vi "Param limits calc.vi"(6 "control":T1={"GAIN"=1.0, "OFFSET"=0.0, "TIME_CONST"=100.0, "MINOFFSET"=2.0, "PVMIN"=0.0, "MINACC"=0.0, "LL"=1.0, "L"=2.0, "H"=6.0, "HH"=7.0, "MAXACC"=9.0, "PVMAX"=10.0, "MAXOFFSET"=2.0, "D"=0.5, "VMAX"=0.0, "TOUT"=1.0, "APERTURE"=0.0} {"APERTURE" min=-100000.0 max=100000.0 step=0.0010000000474974513; "TOUT" min=0.0 max=100000.0 step=1.0; "D" min=-100000.0 max=100000.0 step=0.0010000000474974513; "MAXOFFSET" min=0.0 max=50.0 step=0.0010000000474974513; "PVMAX" min=-100000.0 max=100000.0 step=0.0010000000474974513; "MAXACC" min=-100000.0 max=100000.0 step=0.0010000000474974513; "HH" min=-100000.0 max=100000.0 step=0.0010000000474974513; "H" min=-100000.0 max=100000.0 step=0.0010000000474974513; "L" min=-100000.0 max=100000.0 step=0.0010000000474974513; "LL" min=-100000.0 max=100000.0 step=0.0010000000474974513; "MINACC" min=-100000.0 max=100000.0 step=0.0010000000474974513; "PVMIN" min=-100000.0 max=100000.0 step=0.0010000000474974513; "MINOFFSET" min=0.0 max=50.0 step=0.0010000000474974513; "TIME_CONST" min=1.0 max=100000.0 step=1.0; "OFFSET" min=-100000.0 max=100000.0 step=0.0010000000474974513; "GAIN" min=0.0010000000474974513 max=1000.0 step=0.0010000000474974513}, 7 "PV":dbl step=0.009999999776482582) -> (0 "block":u32 format="%09b", 1 "Off":u32 format="%09b", 2 "On":u32 format="%09b", 3 "PVOUT":dbl format="%#_3g")   [LabVIEW 2019, in "Inputs.lvlib"]
uses:
  Inputs.lvlib
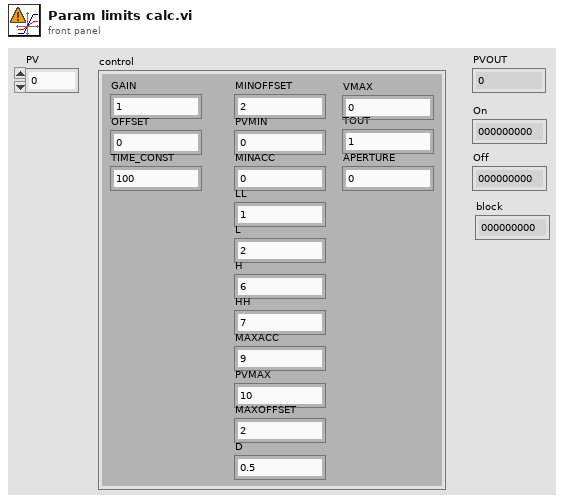
[diagram p1: front panel]
types:
  T1 = cluster{"GAIN":dbl, "OFFSET":dbl, "TIME_CONST":dbl, "MINOFFSET":dbl, "PVMIN":dbl, "MINACC":dbl, "LL":dbl, "L":dbl, "H":dbl, "HH":dbl, "MAXACC":dbl, "PVMAX":dbl, "MAXOFFSET":dbl, "D":dbl, "VMAX":dbl, "TOUT":dbl, "APERTURE":dbl}
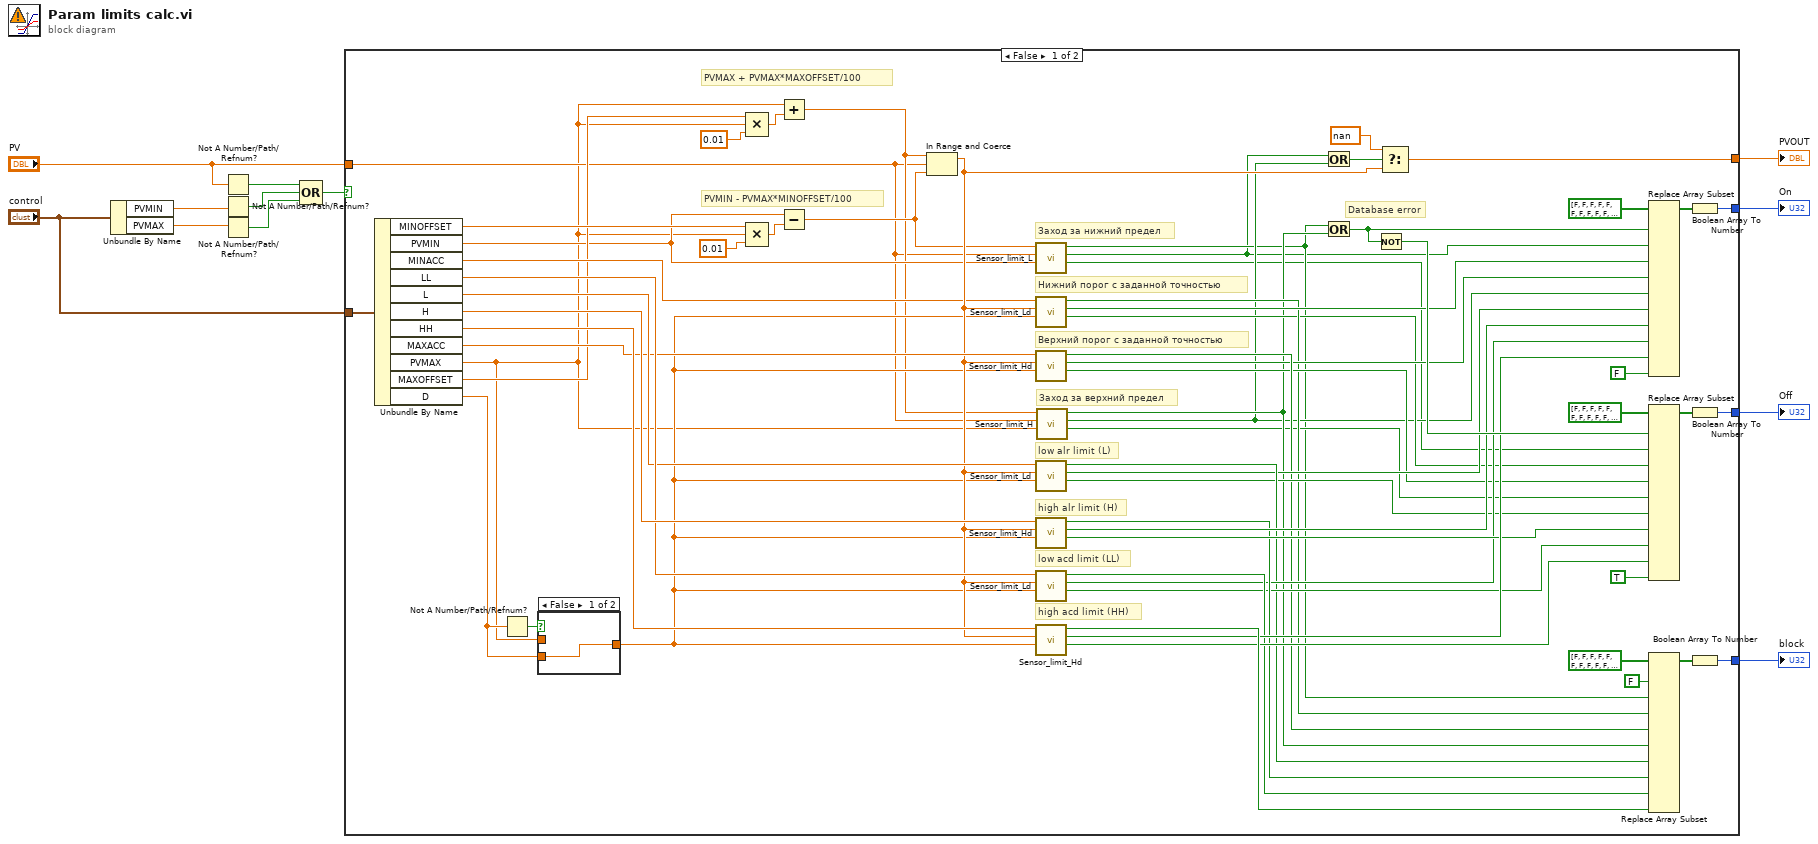
[diagram p0: block diagram]
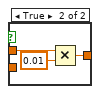
[diagram p2: hidden frame]
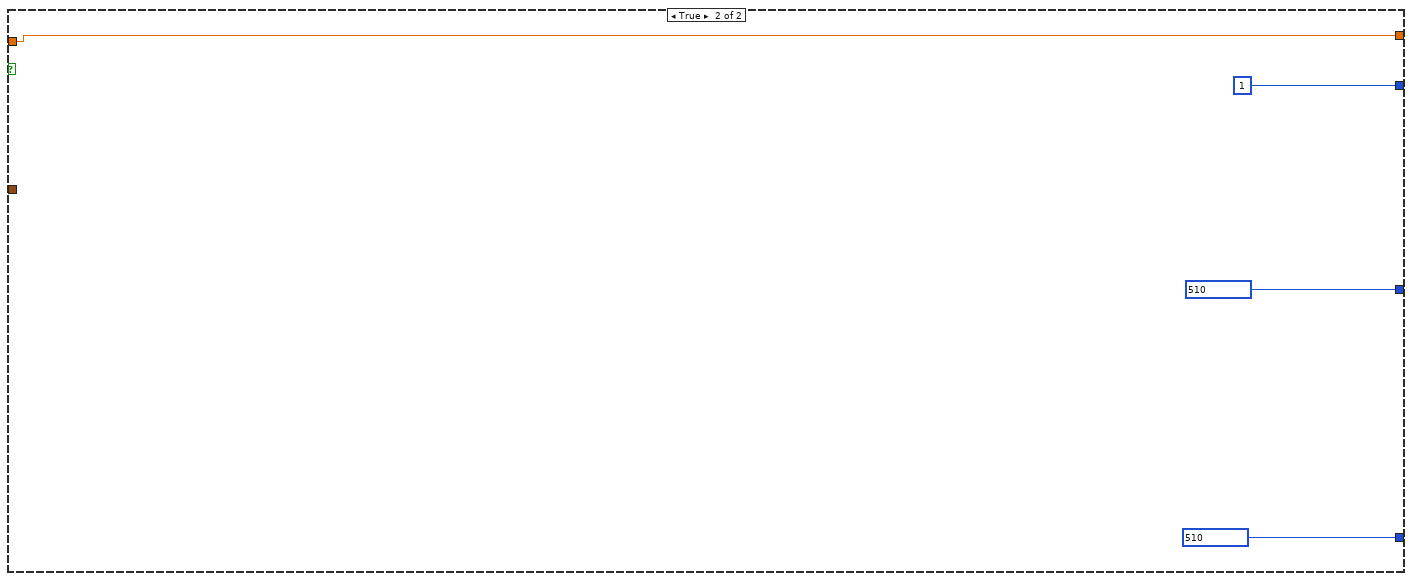
[diagram p3: hidden frame]
diagram:
  n1 = Unbundle By Name("control") -> ("PVMIN"=w10:dbl, "PVMAX"=w9:dbl)
  n2 = Not A Number/Path/Refnum?(number/path/refnum="PV") -> (NaN/Path/Refnum?=w8:bool)
  n3 = Not A Number/Path/Refnum?(number/path/refnum=w10) -> (NaN/Path/Refnum?=w12:bool)
  n4 = Not A Number/Path/Refnum?(number/path/refnum=w9) -> (NaN/Path/Refnum?=w11:bool)
  n5 = Compound Arithmetic op=OR(w8, w12, w11) -> (w6:bool)
  n6 = case shown="False" w6 {
    tunnel: [w72 w83] -> w4
    tunnel: "PV" -> [w17 w83]
    tunnel: [w62 u32 1] -> w3
    tunnel: [w65 u32 510] -> w2
    tunnel: "control" -> [w75 _]
    tunnel: [w74 u32 510] -> w1
    frame False {
      # "Database error"
      # "Верхний порог с заданной точностью"
      # "high acd limit (HH)"
      # "high alr limit (H)"
      # "low acd limit (LL)"
      # "low alr limit (L)"
      # "Заход за верхний предел"
      # "Нижний порог с заданной точностью"
      # "Заход за нижний предел"
      # "PVMIN - PVMAX*MINOFFSET/100"
      # "PVMAX + PVMAX*MAXOFFSET/100"
      n7 = Unbundle By Name(w75) -> ("MINOFFSET"=w60:dbl, "PVMIN"=w20:dbl, "MINACC"=w30:dbl, "LL"=w46:dbl, "L"=w42:dbl, "H"=w50:dbl, "HH"=w54:dbl, "MAXACC"=w36:dbl, "PVMAX"=w13:dbl, "MAXOFFSET"=w23:dbl, "D"=w38:dbl)
      n8 = Not A Number/Path/Refnum?(number/path/refnum=w38) -> (NaN/Path/Refnum?=w37:bool)
      n9 = case shown="False" w37 {
        tunnel: w13 -> [_ w78]
        tunnel: [w76 w77] -> w31
        tunnel: w38 -> [w76 _]
        frame False {
        }
        frame True {
          n10 = Multiply(x=w78, y=0.01) -> (x*y=w77:dbl)
        }
      }
      n11 = Compound Arithmetic op=MULTIPLY(w23, w13, 0.01 ("value")) -> (w21:dbl)
      n12 = Compound Arithmetic op=MULTIPLY(w60, w13, 0.01 ("value")) -> (w59:dbl)
      n13 = Add(x=w13, y=w21) -> (x+y=w18:dbl)
      n14 = Subtract(x=w20, y=w59) -> (x-y=w19:dbl)
      n15 = In Range and Coerce(upper limit=w18, x=w17, lower limit=w19) -> (coerced(x)=w32:dbl)  [unwired: 1 out]
      n16 = call "Sensor_limit_L.vi"("Off L"=w20, "PV"=w17, "Limit L"=w19) -> ("Off"=w14:bool, "On"=w15:bool, "NaN"=w16:bool)  [unwired: 6 in]
      n17 = call "Sensor_limit_Ld.vi"("d"=w31, "PV"=w32, "Limit L"=w30) -> ("Off"=w27:bool, "On"=w29:bool, "NaN"=w28:bool)  [unwired: 6 in]
      n18 = call "Sensor_limit_Hd.vi"("d"=w31, "PV"=w32, "Limit H"=w36) -> ("Off"=w33:bool, "On"=w34:bool, "NaN"=w35:bool)  [unwired: 6 in]
      n19 = call "Sensor_limit_Ld.vi"("d"=w31, "PV"=w32, "Limit L"=w42) -> ("Off"=w39:bool, "On"=w40:bool, "NaN"=w41:bool)  [unwired: 6 in]
      n20 = call "Sensor_limit_Hd.vi"("d"=w31, "PV"=w32, "Limit H"=w50) -> ("Off"=w48:bool, "On"=w49:bool, "NaN"=w47:bool)  [unwired: 6 in]
      n21 = call "Sensor_limit_Ld.vi"("d"=w31, "PV"=w32, "Limit L"=w46) -> ("Off"=w43:bool, "On"=w44:bool, "NaN"=w45:bool)  [unwired: 6 in]
      n22 = call "Sensor_limit_Hd.vi"("d"=w31, "PV"=w32, "Limit H"=w54) -> ("Off"=w51:bool, "On"=w52:bool, "NaN"=w53:bool)  [unwired: 6 in]
      n23 = call "Sensor_limit_H.vi"("Off H"=w13, "PV"=w17, "Limit H"=w18) -> ("Off"=w24:bool, "On"=w25:bool, "NaN"=w26:bool)  [unwired: 6 in]
      n24 = Or(x=w15, y=w25) -> (x .or. y?=w71:bool)
      n25 = Or(x=w16, y=w26) -> (x .or. y?=w63:bool)
      n26 = Not(x=w63) -> (.not. x?=w66:bool)
      n27 = Select(t=nan, s=w71, f=w32) -> (s? t:f=w72:dbl)
      n28 = Replace Array Subset(array=bool[] [FALSE, FALSE, FALSE, FALSE, FALSE, FALSE, FALSE, FALSE, FALSE, FALSE, FALSE, FALSE, FALSE, FALSE, FALSE, FALSE] ("appended array"), new element #1=w63, new element #2=w15, new element #3=w29, new element #4=w34, new element #5=w25, new element #6=w40, new element #7=w49, new element #8=w44, new element #9=w52, new element #10=FALSE ("new element/subarray")) -> (w64:bool[])  [unwired: 10 in]
      n29 = Replace Array Subset(array=bool[] [FALSE, FALSE, FALSE, FALSE, FALSE, FALSE, FALSE, FALSE, FALSE, FALSE, FALSE, FALSE, FALSE, FALSE, FALSE, FALSE] ("appended array"), new element #1=w66, new element #2=w14, new element #3=w27, new element #4=w33, new element #5=w24, new element #6=w39, new element #7=w48, new element #8=w43, new element #9=w51, new element #10=TRUE ("new element/subarray")) -> (w68:bool[])  [unwired: 10 in]
      n30 = Replace Array Subset(array=bool[] [FALSE, FALSE, FALSE, FALSE, FALSE, FALSE, FALSE, FALSE, FALSE, FALSE, FALSE, FALSE, FALSE, FALSE, FALSE, FALSE] ("appended array"), new element #1=FALSE ("new element/subarray"), new element #2=w16, new element #3=w28, new element #4=w35, new element #5=w26, new element #6=w41, new element #7=w47, new element #8=w45, new element #9=w53) -> (w69:bool[])  [unwired: 9 in]
      n31 = Boolean Array To Number(Boolean array=w64) -> (number=w62:u32)
      n32 = Boolean Array To Number(Boolean array=w68) -> (number=w65:u32)
      n33 = Boolean Array To Number(Boolean array=w69) -> (number=w74:u32)
    }
    frame True {
    }
  }
  "PVOUT" <- w4
  "On" <- w3
  "Off" <- w2
  "block" <- w1
